vi "Filter String_Arrow Key Handler.vi"(9 "Done Ref":refnum<vi>, 10 "Tree Ref Array":refnum<vi>[](array[refnum]), 11 "Filter String Ref":refnum<vi>) -> ()   [LabVIEW 2023]
doc: "Down arrow or tab from filter goes to tree's first selectable item. Up arrow from filter goes to tree's last selectable item."
panel:
  out "Shift":bool
  # "DEBUGGING"
  # "Filter"
  # "Tree"
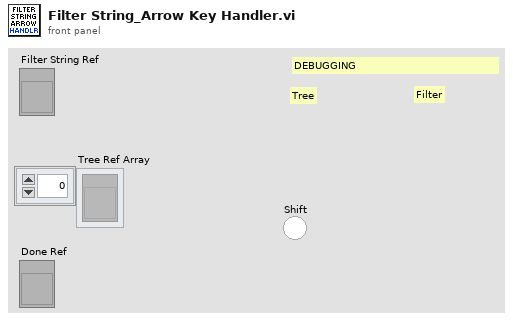
[diagram p1: front panel]
types:
  T1 = typedef "eventvkey.ctl" = enum16{"ASCII", "Enter", "Return", "Shift", "Ctrl", "Alt", "Cmd", "Opt", "Caps", "NumLock", "Clear", "Break", "Up", "Down", "Left", "Right", "Insert", "Delete", "Home", "End", "PageUp", "PageDown", "Escape", "Help", "Pause", "ScrollLock", "F1", "F2", "F3", "F4", "F5", "F6", "F7", "F8", "F9", "F10", "F11", "F12", "F13", "F14", "F15", "F16", "F17", "F18", "F19", "F20", "F21", "F22", "F23", "F24", "Play", "VolumeUp", "VolumeDown", "Mute", "Two Byte Char"}
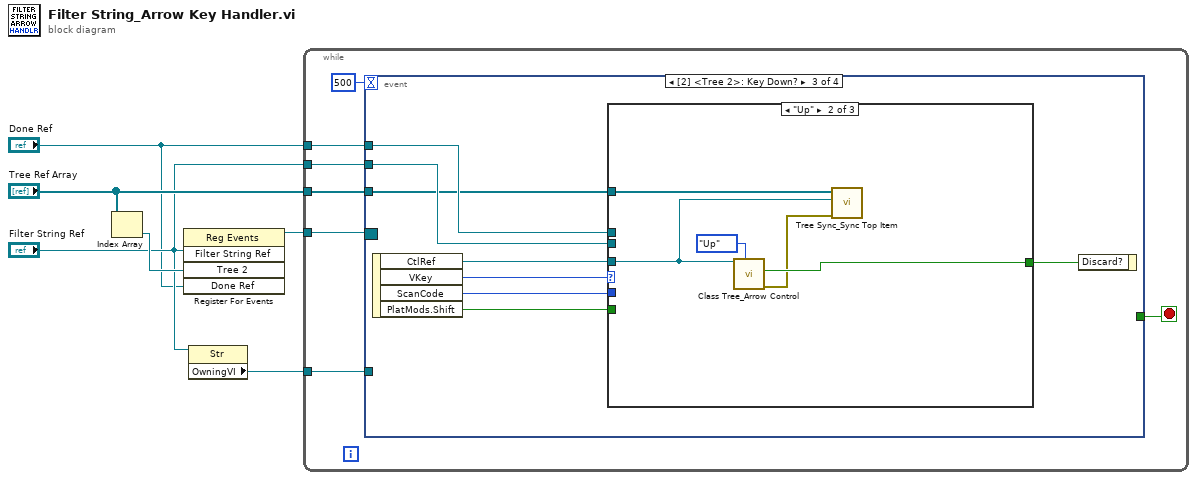
[diagram p0: block diagram]
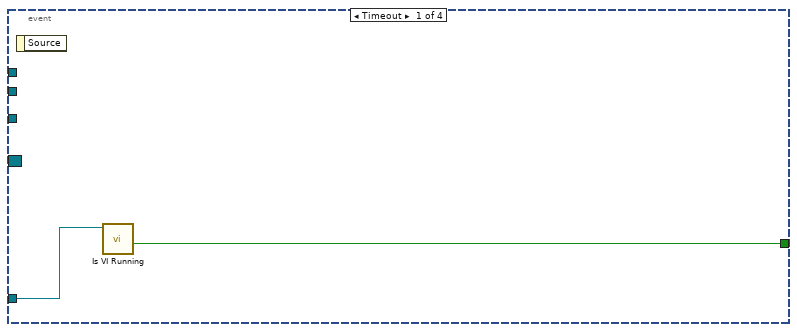
[diagram p2: hidden frame]
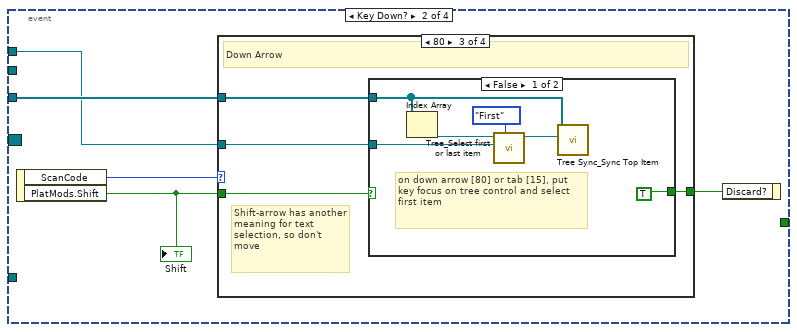
[diagram p3: hidden frame]
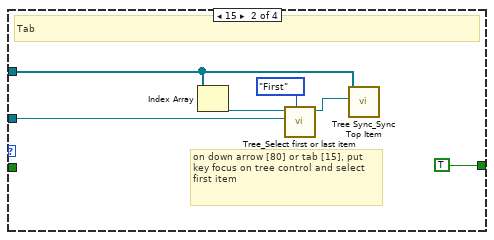
[diagram p5: hidden frame]
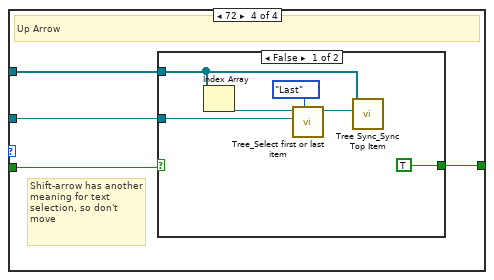
[diagram p7: hidden frame]
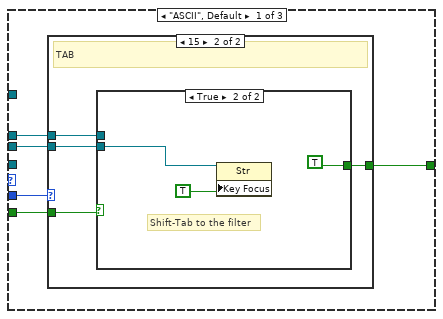
[diagram p9: hidden frame]
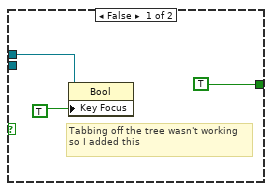
[diagram p11: hidden frame]
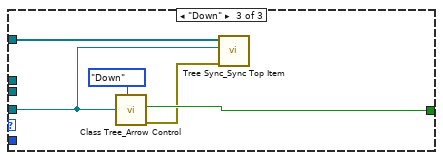
[diagram p12: hidden frame]
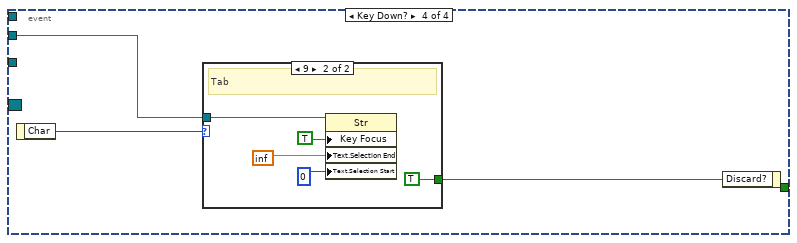
[diagram p13: hidden frame]
diagram:
  n1 = Index Array(array="Tree Ref Array") -> (element=w3:refnum<vi>)  [unwired: 1 in]
  n2 = register-events("Filter String Ref", w3, "Done Ref") -> (reference out=w6:refnum<event-registration>)  [unwired: 2 in, 1 out]
  n3 = property class="Str"(reference="Filter String Ref") -> ("OwningVI"=w5:refnum<vi>)  [unwired: 1 in, 2 out]
  n4 = while {
    tunnel: w6 -> [w11]
    tunnel: w5 -> [w10]
    tunnel: "Tree Ref Array" -> [w9]
    tunnel: "Done Ref" -> [w8]
    tunnel: "Filter String Ref" -> [w7]
    stop <- w13 stop-if-true
    n5 = event shown="[2] <Tree 2>: Key Down?" {
      selector: w11 -> [_ _ _ _]
      dyn-events: _ -> [_ _ _ _]
      timeout: 500 -> [_ _ _ _]
      tunnel: [w14 _ _ _] -> w13
      tunnel: w10 -> [w15 _ _ _]
      tunnel: w9 -> [_ w20 w47 _]
      tunnel: w8 -> [_ w19 w52 _]
      tunnel: w7 -> [_ _ w50 w82]
      event Timeout {
        n6 = event-data() -> ()  [unwired: 1 in, 1 out]
        n7 = call "Is VI Running.vi"("VI in"=w15) -> ("VI Not Running"=w14:bool)  [unwired: 7 in, 3 out]
      }
      event Key Down? {
        n8 = event-data() -> ("ScanCode"=w17:i16, "PlatMods.Shift"=w16:bool)  [unwired: 1 in]
        "Shift" <- w16
        n9 = case shown="80" w17 {
          tunnel: w20 -> [_ w26 w30 w40]
          tunnel: w16 -> [_ _ w29 w39]
          tunnel: w19 -> [_ w25 w28 w38]
          tunnel: [_ TRUE ("Discard?") w27 w37] -> w18
          frame Default {
          }
          frame 15 {
            # "on down arrow [80] or tab [15], put key focus on tree control and select first item"
            # "Tab"
            n10 = Index Array(array=w26) -> (element=w22:refnum<vi>)  [unwired: 1 in]
            n11 = call "Tree_Select first or last item.vi"("Select Item"=enum16{"First", "Last"}."First", "Done Ref"=w25, "Tree Ref"=w22) -> ("Tree Ref Out"=w23:refnum<vi>)  [unwired: 7 in, 1 out]
            n12 = call "Tree Sync_Sync Top Item.vi"("Changed Tree Control Ref"=w23, "All Tree Control Refs"=w26) -> ()  [unwired: 9 in, 1 out]
          }
          frame 80 {
            # "Shift-arrow has another meaning for text selection, so don't move"
            # "Down Arrow"
            n13 = case shown="False" w29 {
              tunnel: w30 -> [w33 _]
              tunnel: w28 -> [w34 _]
              tunnel: [TRUE ("Discard?") _] -> w27
              frame False {
                # "on down arrow [80] or tab [15], put key focus on tree control and select first item"
                n14 = Index Array(array=w33) -> (element=w32:refnum<vi>)  [unwired: 1 in]
                n15 = call "Tree_Select first or last item.vi"("Select Item"=enum16{"First", "Last"}."First", "Done Ref"=w34, "Tree Ref"=w32) -> ("Tree Ref Out"=w35:refnum<vi>)  [unwired: 7 in, 1 out]
                n16 = call "Tree Sync_Sync Top Item.vi"("Changed Tree Control Ref"=w35, "All Tree Control Refs"=w33) -> ()  [unwired: 9 in, 1 out]
              }
              frame True {
              }
            }
          }
          frame 72 {
            # "Shift-arrow has another meaning for text selection, so don't move"
            # "Up Arrow"
            n17 = case shown="False" w39 {
              tunnel: w40 -> [w43 _]
              tunnel: w38 -> [w44 _]
              tunnel: [TRUE ("Discard?") _] -> w37
              frame False {
                n18 = Index Array(array=w43) -> (element=w42:refnum<vi>)  [unwired: 1 in]
                n19 = call "Tree_Select first or last item.vi"("Select Item"=enum16{"First", "Last"}."Last", "Done Ref"=w44, "Tree Ref"=w42) -> ("Tree Ref Out"=w45:refnum<vi>)  [unwired: 7 in, 1 out]
                n20 = call "Tree Sync_Sync Top Item.vi"("Changed Tree Control Ref"=w45, "All Tree Control Refs"=w43) -> ()  [unwired: 9 in, 1 out]
              }
              frame True {
              }
            }
          }
        }
        n21 = event-data("Discard?"=w18) -> ()  [unwired: 1 in, 1 out]
      }
      event Key Down? {
        n22 = event-data() -> ("CtlRef"=w54:refnum<vi>, "VKey"=w51:T1, "ScanCode"=w49:i16, "PlatMods.Shift"=w48:bool)  [unwired: 1 in]
        n23 = case shown="\"Up\"" w51 {
          tunnel: [w59 w73 w79] -> w53
          tunnel: w54 -> [_ w71 w75]
          tunnel: w49 -> [w58 _ _]
          tunnel: w52 -> [w57 _ _]
          tunnel: w48 -> [w56 _ _]
          tunnel: w50 -> [w55 _ _]
          tunnel: w47 -> [_ w72 w76]
          frame "ASCII", Default {
            n24 = case shown="15" w58 {
              tunnel: [_ w63] -> w59
              tunnel: w57 -> [_ w62]
              tunnel: w56 -> [_ w61]
              tunnel: w55 -> [_ w60]
              frame Default {
              }
              frame 15 {
                # "TAB"
                n25 = case shown="True" w61 {
                  tunnel: [TRUE ("discard") TRUE ("discard")] -> w63
                  tunnel: w62 -> [w64 _]
                  tunnel: w60 -> [_ w68]
                  frame False {
                    # "Tabbing off the tree wasn't working so I added this"
                    n26 = property class="Bool"(reference=w64, "Key Focus"=TRUE) -> ()  [unwired: 1 in, 2 out]
                  }
                  frame True {
                    # "Shift-Tab to the filter"
                    n27 = property class="Str"(reference=w68, "Key Focus"=TRUE) -> ()  [unwired: 1 in, 2 out]
                  }
                }
              }
            }
          }
          frame "Up" {
            n28 = call "Class Tree_Arrow Control.vi"("Direction"=enum16{"Down", "Up"}."Up", "Tree ref"=w71) -> ("error out"=w70:errorcluster, "discard"=w73:bool)  [unwired: 8 in]
            n29 = call "Tree Sync_Sync Top Item.vi"("error in"=w70, "Changed Tree Control Ref"=w71, "All Tree Control Refs"=w72) -> ()  [unwired: 8 in, 1 out]
          }
          frame "Down" {
            n30 = call "Class Tree_Arrow Control.vi"("Direction"=enum16{"Down", "Up"}."Down", "Tree ref"=w75) -> ("error out"=w77:errorcluster, "discard"=w79:bool)  [unwired: 8 in]
            n31 = call "Tree Sync_Sync Top Item.vi"("error in"=w77, "Changed Tree Control Ref"=w75, "All Tree Control Refs"=w76) -> ()  [unwired: 8 in, 1 out]
          }
        }
        n32 = event-data("Discard?"=w53) -> ()  [unwired: 1 in, 1 out]
      }
      event Key Down? {
        n33 = event-data() -> ("Char"=w81:i16)  [unwired: 1 in]
        n34 = case shown="9" w81 {
          tunnel: [_ TRUE ("Discard?")] -> w80
          tunnel: w82 -> [_ w83]
          frame 0, Default {
          }
          frame 9 {
            # "Tab"
            n35 = property class="Str"(reference=w83, "Key Focus"=TRUE, "Text.Selection End"=inf, "Text.Selection Start"=u32 0 ("Text.Selection:Start")) -> ()  [unwired: 1 in, 2 out]
          }
        }
        n36 = event-data("Discard?"=w80) -> ()  [unwired: 1 in, 1 out]
      }
    }
  }
